vi "readMatFileToNx1Array.vi"(7 "Path":path, 8 "error in (no error)":errorcluster, 9 "Index of Column":i32[](array[numeric]), 10 "Index of Row":i32[](array[numeric]), 11 "MatOper in":refnum<class "MatOper.lvclass">) -> (0 "error out":errorcluster, 2 "nx1 Array":dbl[][](array[numeric]), 3 "MatOper out":refnum<class "MatOper.lvclass">)   [LabVIEW 2016, in "MatOper.lvclass"]
doc: "Read the 2D matrix file and transform to nx1 array based on the index of row and column."
uses:
  MatOper.lvclass
  getSubArray2D.vi
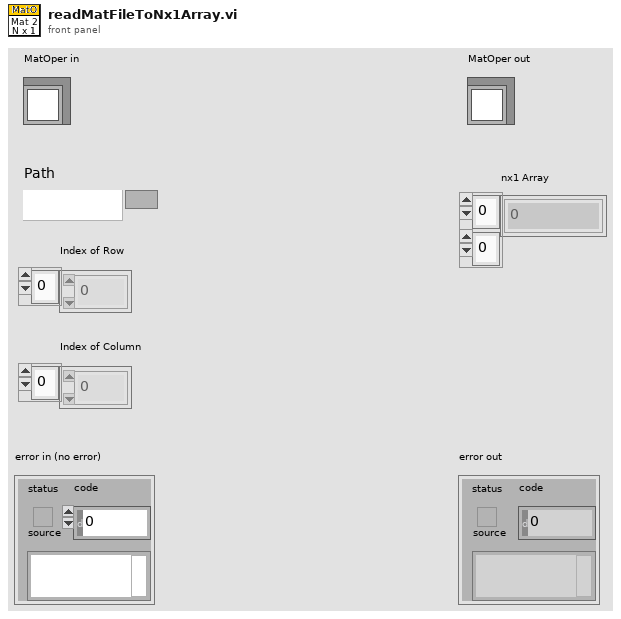
[diagram p1: front panel]
types:
  T1 = cluster{"Index of Row":i32[], "Index of Column":i32[]}
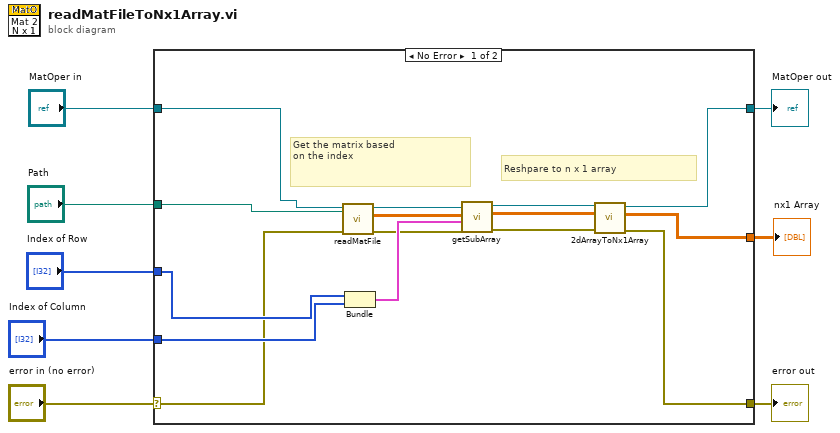
[diagram p0: block diagram]
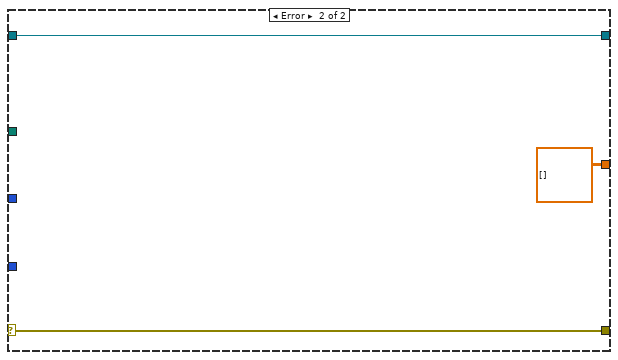
[diagram p2: hidden frame]
diagram:
  n1 = case shown="No Error" "error in (no error)" {
    selector: "error in (no error)" -> [w15 w26]
    tunnel: [w13 w26] -> w7
    tunnel: [w9 w25] -> w5
    tunnel: "MatOper in" -> [w12 w25]
    tunnel: [w19 dbl[][] [] ("nx1 Array")] -> w4
    tunnel: "Path" -> [w18 _]
    tunnel: "Index of Row" -> [w17 _]
    tunnel: "Index of Column" -> [w16 _]
    frame No Error {
      # "Get the matrix based \non the index"
      # "Reshpare to n x 1 array"
      n2 = call "readMatFile.vi"("Path"=w18, "error in (no error)"=w15, "MatOper in"=w12) -> ("error out"=w20:errorcluster, "Matrix"=w21:dbl[][], "MatOper out"=w11:refnum<class "MatOper.lvclass">)  [unwired: 6 in]
      n3 = Bundle("Index of Row"=w17, "Index of Column"=w16) -> (w23:T1)  [unwired: 1 in]
      n4 = call-poly "getSubArray.vi"("error in (no error)"=w20, "Index Array Cluster"=w23, "2D Array"=w21, "MatOper in"=w11) -> ("error out"=w14:errorcluster, "Sub-Array"=w22:dbl[][], "MatOper out"=w10:refnum<class "MatOper.lvclass">)  [unwired: 5 in]
      n5 = call "2dArrayToNx1Array.vi"("error in (no error)"=w14, "2D Array"=w22, "MatOper in"=w10) -> ("error out"=w13:errorcluster, "nx1 Array"=w19:dbl[][], "MatOper out"=w9:refnum<class "MatOper.lvclass">)  [unwired: 6 in]
    }
    frame Error {
    }
  }
  "error out" <- w7
  "MatOper out" <- w5
  "nx1 Array" <- w4
